vi "SVL Decimated Exp Avg Level (resampled) (1 Ch).vi"(6 "restart averaging (F)":bool, 7 "decimation factor":i32=-1, 8 "error in (no error)":errorcluster, 9 "exponential weighting":dbl=1.0 format="%.2f", 10 "even-angle channel info":T1={"channel name"="", "description"="", " channel info"={"sensor sensitivity"=1000.0, "engineering units"=1, "dB reference"=1.0, "custom label"="EU", "weighting filter"=0, "pregain"=0.0}} {"channel info"."pregain" format="%.2f"; "channel info"."weighting filter" items=["Linear", "A-weighting", "B-weighting", "C-weighting", "ITU-R 468-4", "Dolby", "CCITT", "C-message", "Wb", "Wc", "Wd", "We", "Wf", "Wh", "Wj", "Wk", "Wm", "AES17 20 kHz lowpass", "AES17 40 kHz lowpass", "AES17 20 kHz highpass", "AES17 40 kHz highpass"]; "channel info"."dB reference" format="%^.1e"; "channel info"."engineering units" items=["custom..."=0, "V"=1, "A"=21, "C"=30, "pC"=31, "s"=32, "-"=29, "Pa"=2, "N"=20, "g"=3, "m/s^2"=4, "m/s"=5, "m"=6, "mm/s"=12, "mm"=13, "micron/s"=14, "micron"=15, "in/s^2"=7, "in/s"=8, "in"=9, "mil/s"=10, "mil"=11, "rad/s^2"=16, "rad/s"=17, "rad"=18, "deg/s^2"=26, "deg/s"=27, "deg"=28, "RPM"=22, "cycle/s^2"=23, "Hz"=24, "cycle"=25, "strain"=19]; "channel info"."sensor sensitivity" format="%#_5f"}, 11 "even-angle signal [EU]":T5 {"even-angle signal" format="%.2f"; "dr" format="%.2f"; "r0" format="%.2f"}) -> (0 "error out":errorcluster, 2 "unit label":string, 3 "decimated exp avg level [EU rms]":cluster{"r0":dbl, "dr":dbl, "level":dbl[]} {"level" format="%.2f"; "dr" format="%.2f"; "r0" format="%.2f"}, 5 "actual decimation factor":i32=1 min=1 step=1)   [LabVIEW 2017, in "SoundVib_VibrationLevel.lvlib"]
doc: "Computes the exponential average level of <B>scaled signal [EU]</B> or <B>even-angle signal [EU]</B> and then decimates the level signal by <B>decimation factor</B>. <B>scaled signal [EU]</B> should have a zero DC component. You can attenuate the DC component with hardware AC-coupling filters and with software high-pass filters. Wire data to the <B>scaled signal [EU]</B> input to determine the polymorphic instance to use or manually select the instance."
uses:
  <vilib>/addons/Sound and Vibration/svt_Level/SoundVib_VibrationLevel.lvlib
  <vilib>/addons/_NISVFA/_Shared subVIs/Controls/svc_Resampled Channel Info.ctl
  <vilib>/addons/_NISVFA/_Shared subVIs/Controls/svc_Channel Info.ctl
  <vilib>/addons/_NISVFA/_Shared subVIs/Controls/svc_Engineering Units Text Ring.ctl
  <vilib>/addons/_NISVFA/_Shared subVIs/Controls/svc_Weighting Filter Text Ring.ctl
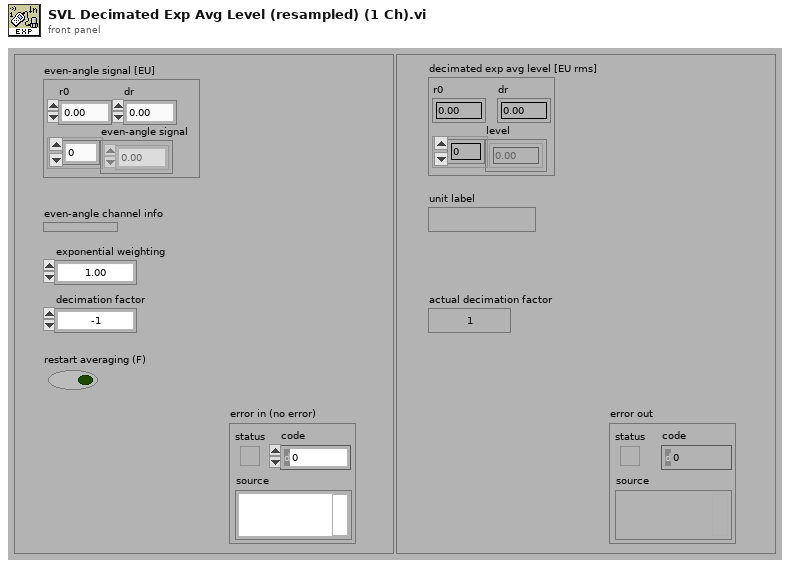
[diagram p1: front panel]
types:
  T1 = typedef "svc_Resampled Channel Info.ctl" = cluster{"channel name":string, "description":string, " channel info":T2}
  T2 = typedef "svc_Channel Info.ctl" = cluster{"sensor sensitivity":dbl, "engineering units":T3, "dB reference":dbl, "custom label":string, "weighting filter":T4, "pregain":dbl}
  T3 = typedef "svc_Engineering Units Text Ring.ctl" = u16
  T4 = typedef "svc_Weighting Filter Text Ring.ctl" = u16
  T5 = cluster{"r0":dbl, "dr":dbl, "even-angle signal":dbl[]}
  T6 = enum16{"RMS", "Running RMS", "Exp avg  ", "Dec exp avg ", "Peak", "Crest"}
  T7 = cluster{"r0":dbl, "dr":dbl, "even angle signal":dbl[]}
  T8 = enum16{"Reset filter", "Restart averaging", "Continue processing"}
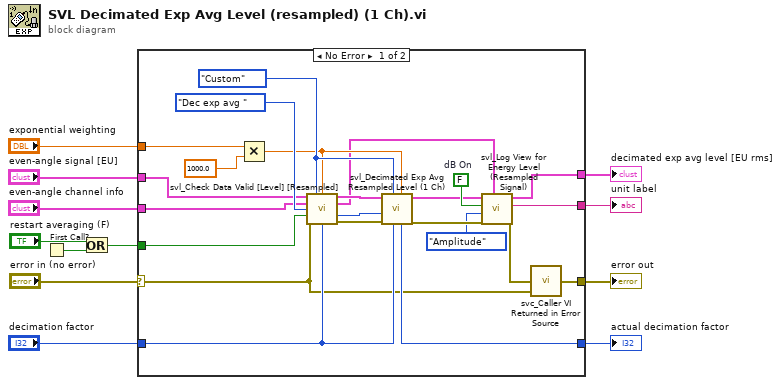
[diagram p0: block diagram]
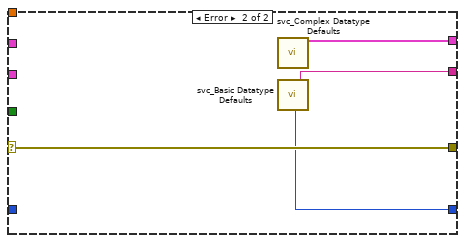
[diagram p2: hidden frame]
diagram:
  n1 = First Call?() -> (First Call?: T/F=w7:bool)
  n2 = Or(x="restart averaging (F)", y=w7) -> (x .or. y?=w6:bool)
  n3 = case shown="No Error" "error in (no error)" {
    tunnel: [w14 w36] -> w12
    tunnel: [w26 w39] -> w11
    tunnel: [w31 w37] -> w10
    tunnel: "even-angle signal [EU]" -> [w17 _]
    tunnel: w6 -> [w25 _]
    tunnel: "exponential weighting" -> [w20 _]
    tunnel: "decimation factor" -> [w24 _]
    tunnel: [w27 w38] -> w3
    selector: "error in (no error)" -> [w13 w39]
    tunnel: "even-angle channel info" -> [w16 _]
    frame No Error {
      w22 = enum16{"Slow", "Fast", "Impulse", "Custom"}."Custom" ("exponential mode")
      w32 = FALSE  # dB On
      n4 = Multiply(x=w20, y=1000.0) -> (x*y=w19:dbl)
      n5 = call <vilib>:"svl_Check Data Valid [Level] [Resampled].vi"("even angle signal"=w17, "exponential mode"=w22, "time constant [ms]"=w19, "even angle channel info"=w16, "Level Analysis"=T6."Dec exp avg ", "restart averaging (F)"=w25, "error in (no error)"=w13, "decimation factor"=w24) -> ("dup even angle signal"=w18:T7, "dup even angle channel info"=w15:T1, "processing state"=w28:T8, "error out"=w35:errorcluster)  [unwired: 4 in]
      n6 = call <vilib>:"svl_Decimated Exp Avg Resampled Level (1 Ch).vi"("time constant [ms]"=w19, "decimation factor"=w24, "exponential mode"=w22, "error in (no error)"=w35, "processing state"=w28, "even angle signal"=w18) -> ("error out"=w34:errorcluster, "even angle signal"=w30:T7, "actual decimation factor"=w27:i32)  [unwired: 2 in, 1 out]
      n7 = call <vilib>:"svl_Log View for Energy Level (Resampled Signal).vi"("resampled channel info"=w15, "error in (no error)"=w34, "view mode"=enum16{"Power", "Amplitude"}."Amplitude", "dB On (T)"=w32, "even angle signal"=w30) -> ("error out"=w33:errorcluster, "unit label"=w31:string, "even angle signal"=w14:T7)  [unwired: 4 in]
      n8 = call <vilib>:"svc_Caller VI Returned in Error Source.vi"("warning input to caller"=w13, "error in (no error)"=w33) -> ("error out"=w26:errorcluster)  [unwired: 3 in]
    }
    frame Error {
      n9 = call <vilib>:"svc_Complex Datatype Defaults.vi"() -> ("empty spectrum"=w36:cluster{"f0":dbl, "df":dbl, "magnitude":dbl[]})  [unwired: 11 in, 8 out]
      n10 = call <vilib>:"svc_Basic Datatype Defaults.vi"() -> ("zero I32"=w38:i32, "empty string"=w37:string)  [unwired: 7 in, 11 out]
    }
  }
  "unit label" <- w10
  "decimated exp avg level [EU rms]" <- w12
  "error out" <- w11
  "actual decimation factor" <- w3
